vi "lv_icon.vi"(8 "error in (no error)":errorcluster, 9 "BW icon in":T1, 10 "Color icon in":T1, 11 "Icon editor default plugin in":refnum<class "IconEditorDefaultPlugin.lvclass">) -> (0 "error out":errorcluster, 1 "BW icon out":T1, 2 "Color icon out":T1, 3 "_Icon editor default plugin out":refnum<class "IconEditorDefaultPlugin.lvclass">, 4 "Error code out":i32)   [LabVIEW 2021, in "IconEditorDefaultPlugin.lvlib" / "IconEditorDefaultPlugin.lvclass"]
uses:
  <resource>/plugins/NIIconEditor/UI/Default/IconEditorDefaultPlugin.lvclass
  <vilib>/picture/picture.llb/imagedata.ctl
  <resource>/plugins/NIIconEditor/UI/Default/IconEditorDefaultPlugin.lvclass/IconEditorDefaultPlugin.ctl
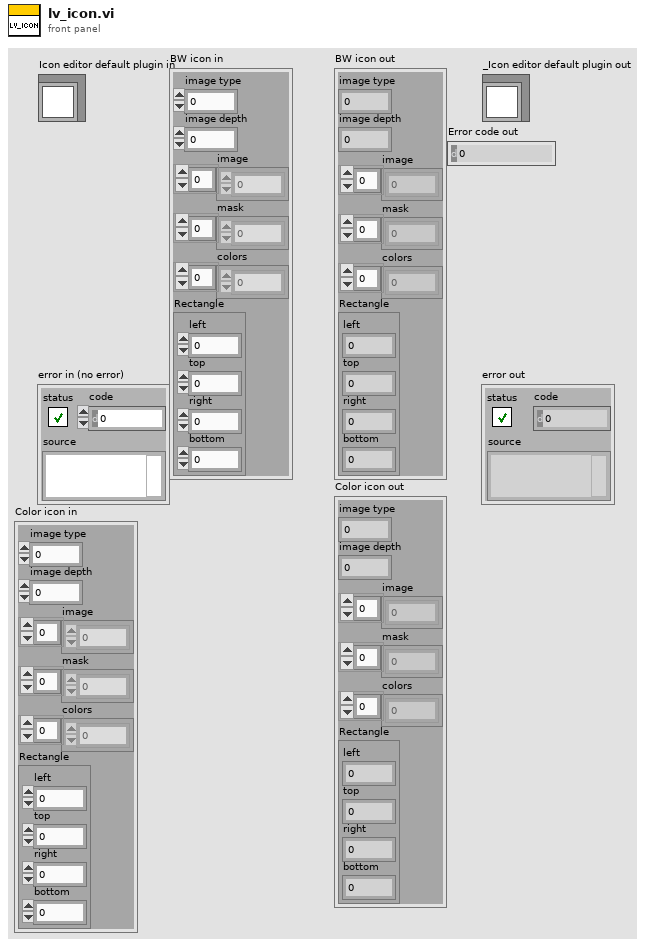
[diagram p1: front panel]
types:
  T1 = typedef "imagedata.ctl" = cluster{"image type":i32, "image depth":i32, "image":u8[], "mask":u8[], "colors":u32[], "Rectangle":cluster{"left":i16, "top":i16, "right":i16, "bottom":i16}}
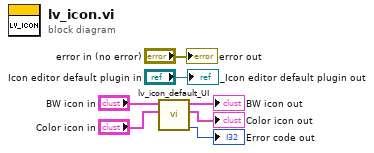
[diagram p0: block diagram]
diagram:
  n1 = call <resource>:"lv_icon_default_UI.vi"("Color icon in"="Color icon in", "BW icon in"="BW icon in") -> ("Error code out"=→"Error code out":i32, "Color icon out"=→"Color icon out":T1, "BW icon out"=→"BW icon out":T1)  [unwired: 7 in]
  "error out" <- "error in (no error)"
  "_Icon editor default plugin out" <- "Icon editor default plugin in"
